vi "switchSolenoid_topLvl.vi"(5 "which manipulator":T1(ring), 8 "error in (no error)":errorcluster, 10 "solenoidSwitch (T:atm; F: Reg)":bool, 11 "Pressure box control in":T2) -> (0 "error out":errorcluster, 3 "Pressure box control out":T2)   [LabVIEW 2019]
uses:
  controls/pressure_box_control.ctl
  controls/pressure_box_type.ctl
  controls/proportionAir_cmds.ctl
  controls/arduino_pressure_setting.ctl
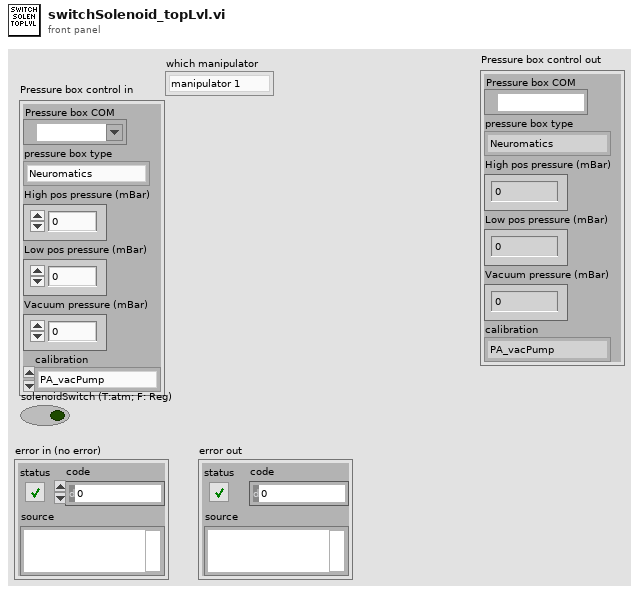
[diagram p1: front panel]
types:
  T1 = enum16{"manipulator 1", "manipulator 2", "manipulator 3", "manipulator 4"}
  T2 = typedef "pressure_box_control.ctl" = cluster{"Pressure box COM":refnum<visa-resource-name>, "pressure box type":T3, "High pos pressure (mBar)":dbl, "Low pos pressure (mBar)":dbl, "Vacuum pressure (mBar)":dbl, "calibration":enum16{"PA_vacPump", "PA_venturi", "Neuromatics", "ilyaRig", "mightenRig"}}
  T3 = typedef "pressure_box_type.ctl" = enum16{"Neuromatics", "ProportionAir", "Demo box", "N-ProportionAir"}
  T4 = typedef "proportionAir_cmds.ctl" = enum16{"Set P", "Switch to Atm", "Switch to Regulator", "Pulse", "WC"}
  T5 = typedef "arduino_pressure_setting.ctl" = enum16{"High Positive Pressure", "Low Positive Pressure", "Atmospheric Pressure", "Low Vacuum", "High Vacuum", "Break In", "Puff"}
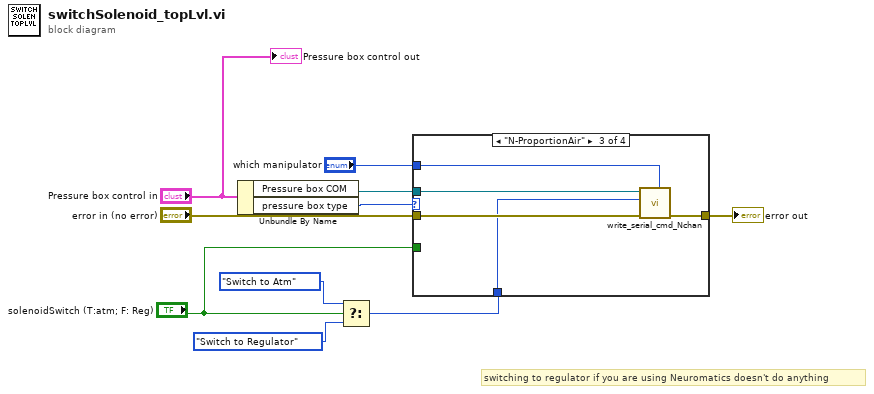
[diagram p0: block diagram]
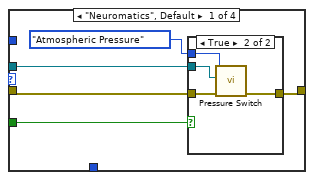
[diagram p2: hidden frame]
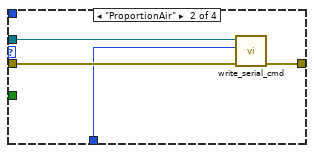
[diagram p4: hidden frame]
diagram:
  # "switching to regulator if you are using Neuromatics doesn't do anything"
  n1 = Unbundle By Name("Pressure box control in") -> ("Pressure box COM"=w8:refnum<visa-resource-name>, "pressure box type"=w9:T3)
  n2 = Select(t=proportionAir_cmds."Switch to Atm" ("pressure command"), s="solenoidSwitch (T:atm; F: Reg)", f=proportionAir_cmds."Switch to Regulator" ("pressure command")) -> (s? t:f=w3:T4)
  n3 = case shown="\"N-ProportionAir\"" w9 {
    tunnel: "error in (no error)" -> [w13 w24 w29 w30]
    tunnel: [w14 w23 w28 w30] -> w7
    tunnel: w8 -> [w15 w22 w27 _]
    tunnel: w3 -> [_ w21 w26 _]
    tunnel: "solenoidSwitch (T:atm; F: Reg)" -> [w12 _ _ _]
    tunnel: "which manipulator" -> [_ _ w25 _]
    frame "Neuromatics", Default {
      n4 = case shown="True" w12 {
        tunnel: w15 -> [_ w20]
        tunnel: [w16 w19] -> w14
        tunnel: w13 -> [w16 w18]
        tunnel: arduino_pressure_setting."Atmospheric Pressure" ("t") -> [_ w17]
        frame False {
        }
        frame True {
          n5 = call "Pressure Switch.vi"("error in"=w18, "Pressure Box COM"=w20, "arduino pressure setting"=w17) -> ("error out"=w19:errorcluster)  [unwired: 7 in, 1 out]
        }
      }
    }
    frame "ProportionAir" {
      n6 = call "write_serial_cmd.vi"("error in"=w24, "pressure command"=w21, "Pressure Box COM"=w22) -> ("error out"=w23:errorcluster)  [unwired: 7 in, 1 out]
    }
    frame "N-ProportionAir" {
      n7 = call "write_serial_cmd_Nchan.vi"("which manipulator"=w25, "error in"=w29, "pressure command"=w26, "Pressure Box COM"=w27) -> ("error out"=w28:errorcluster)  [unwired: 6 in, 1 out]
    }
    frame "Demo box" {
    }
  }
  "error out" <- w7
  "Pressure box control out" <- "Pressure box control in"
